vi "BNO055 Read AMG.vi"(8 "error in (no error)":errorcluster, 9 "BNO055 Config Options":T1={"I2C"={"Slave Address"=72, "Channel"=1}, "ADC"={"Channel"=4, "Expected Range (Programmable Gain Amplifier)"=0, "Sampling Mode"=1, "Sampling Rate"=4, "Comparator Mode"=1, "Comparator Polarity"=1, "Latching Comparator"=1, "Comparator Queue & Disable"=3}} {"ADC"."Comparator Queue & Disable" items=["Assert after one conversion", "Assert after two conversions", "Assert after four conversions", "Comparator disabled"]; "ADC"."Latching Comparator" items=["Non-latching", "Latching"]; "ADC"."Comparator Polarity" items=["Active Low", "Active High"]; "ADC"."Comparator Mode" items=["Traditional Comparator w/ hysteresis", "Window Comparator"]; "ADC"."Sampling Rate" items=["128SPS", "250SPS", "490SPS", "920SPS", "1600SPS", "2400SPS", "3300SPS"]; "ADC"."Sampling Mode" items=["Continuous Conversion", "Single-shot (Low Power)"]; "ADC"."Expected Range (Programmable Gain Amplifier)" items=["+/-6.144V", "+/-4.096V", "+/-2.048V", "+/-1.024V", "+/-0.512V", "+/-0.256V"]; "ADC"."Channel" items=["Differential: Ch 0&1", "Differential: Ch 0&3", "Differential: Ch 1&3", "Differential: Ch 2&3", "Single Ended: Ch 0", "Single Ended: Ch 1", "Single Ended: Ch 2", "Single Ended: Ch 3"]; "I2C"."Slave Address" format="%.0x"}, 11 "LINX Resource in":T3) -> (0 "error out":errorcluster, 1 "BNO055 Config Options":T1={"I2C"={"Slave Address"=72, "Channel"=1}, "ADC"={"Channel"=4, "Expected Range (Programmable Gain Amplifier)"=0, "Sampling Mode"=1, "Sampling Rate"=4, "Comparator Mode"=1, "Comparator Polarity"=1, "Latching Comparator"=1, "Comparator Queue & Disable"=3}} {"ADC"."Comparator Queue & Disable" items=["Assert after one conversion", "Assert after two conversions", "Assert after four conversions", "Comparator disabled"]; "ADC"."Latching Comparator" items=["Non-latching", "Latching"]; "ADC"."Comparator Polarity" items=["Active Low", "Active High"]; "ADC"."Comparator Mode" items=["Traditional Comparator w/ hysteresis", "Window Comparator"]; "ADC"."Sampling Rate" items=["128SPS", "250SPS", "490SPS", "920SPS", "1600SPS", "2400SPS", "3300SPS"]; "ADC"."Sampling Mode" items=["Continuous Conversion", "Single-shot (Low Power)"]; "ADC"."Expected Range (Programmable Gain Amplifier)" items=["+/-6.144V", "+/-4.096V", "+/-2.048V", "+/-1.024V", "+/-0.512V", "+/-0.256V"]; "ADC"."Channel" items=["Differential: Ch 0&1", "Differential: Ch 0&3", "Differential: Ch 1&3", "Differential: Ch 2&3", "Single Ended: Ch 0", "Single Ended: Ch 1", "Single Ended: Ch 2", "Single Ended: Ch 3"]; "I2C"."Slave Address" format="%.0x"}, 2 "IMU":T2 {"Gyroscope"."Z" scale=-45.0..45.0; "Gyroscope"."Y" scale=-45.0..45.0; "Gyroscope"."X" scale=-45.0..45.0; "Magnetometer"."Z" scale=-2500.0..2500.0; "Magnetometer"."Y" scale=-2500.0..2500.0; "Magnetometer"."X" scale=-2500.0..2500.0; "Accelerometer"."Z" scale=-5.0..5.0; "Accelerometer"."Y" scale=-5.0..5.0; "Accelerometer"."X" scale=-5.0..5.0}, 3 "LINX Resource":T3)   [LabVIEW 2014]
uses:
  <vilib>/MakerHub/LINX/Private/Type Defs/LINX Ref.ctl
  <vilib>/MakerHub/LINX/Private/Type Defs/Platform.ctl
  <vilib>/MakerHub/LINX/Private/Type Defs/Interface.ctl
  <vilib>/MakerHub/LINX/Private/Device/Type Defs/LINX Device Config.ctl
  <vilib>/MakerHub/LINX/Private/Device/Type Defs/TCP Config.ctl
  <vilib>/MakerHub/LINX/Private/Device/Type Defs/Channels.ctl
  BNO055 Config Options.ctl
  IMU Control.ctl
  <vilib>/MakerHub/LINX/LMH-LINX.lvlib
  <vilib>/MakerHub/LINX/Private/Device/Device.lvlib
panel:
  out "Array":u32[](array[numeric])
  out "Data out":u8[](array[numeric])
  out "Data":u8[](array[numeric])
  # "NOT DONE\nYET!"
  # "NOT DONE\nYET!"
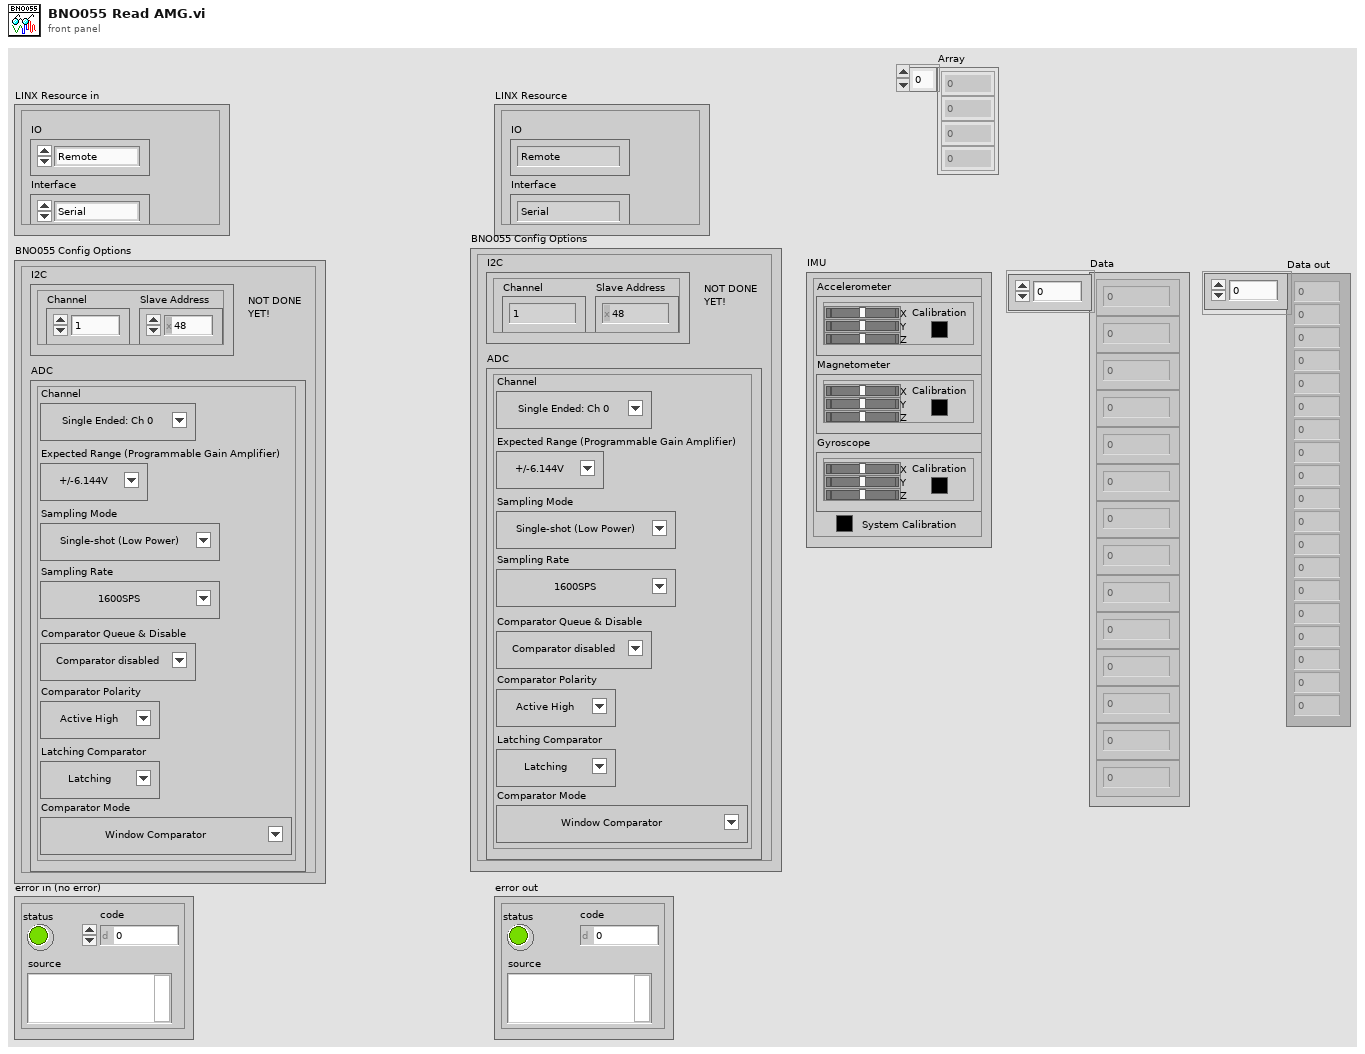
[diagram p1: front panel]
types:
  T1 = typedef "BNO055 Config Options.ctl" = cluster{"I2C":cluster{"Slave Address":u8, "Channel":u8}, "ADC":cluster{"Channel":u8, "Expected Range (Programmable Gain Amplifier)":u8, "Sampling Mode":u8, "Sampling Rate":u8, "Comparator Mode":u8, "Comparator Polarity":u8, "Latching Comparator":u8, "Comparator Queue & Disable":u8}}
  T2 = typedef "IMU Control.ctl" = cluster{"Accelerometer":cluster{"X":dbl, "Y":dbl, "Z":dbl, "Calibration":u32}, "Magnetometer":cluster{"X":dbl, "Y":dbl, "Z":dbl, "Calibration":u32}, "Gyroscope":cluster{"X":dbl, "Y":dbl, "Z":dbl, "Calibration":u32}, "System Calibration":u32}
  T3 = typedef "LMH-LINX.lvlib/LINX Ref.ctl" = cluster{"IO":T4, "Interface":T5, "LINX Device Config":T6}
  T4 = typedef "LMH-LINX.lvlib/Platform.ctl" = enum16{"Remote", "Local"}
  T5 = typedef "LMH-LINX.lvlib/Interface.ctl" = enum16{"Serial", "TCP"}
  T6 = typedef "LMH-LINX.lvlib/Device.lvlib/LINX Device Config.ctl" = cluster{"Interface":T5, "COM Port":refnum<visa-resource-name>, "TCP Configuration":T7, "Device Family":u8, "Device ID":u8, "Device Name":string, "TCP Ref":refnum<k5>, "Channels":T8}
  T7 = typedef "LMH-LINX.lvlib/Device.lvlib/TCP Config.ctl" = cluster{"IP Address":string, "Port":u16}
  T8 = typedef "LMH-LINX.lvlib/Channels.ctl" = cluster{"DI":u8[], "DO":u8[], "AI":u8[], "AO":u8[], "PWM":u8[], "QE":u8[], "UART":u8[], "I2C 2":u8[], "SPI":u8[], "CAN":u8[], "Servo":u8[], "AI Ref (V)":dbl, "AI Resolution (Bits)":u8, "AO Ref (V)":dbl, "AO Resolution (Bits)":u8}
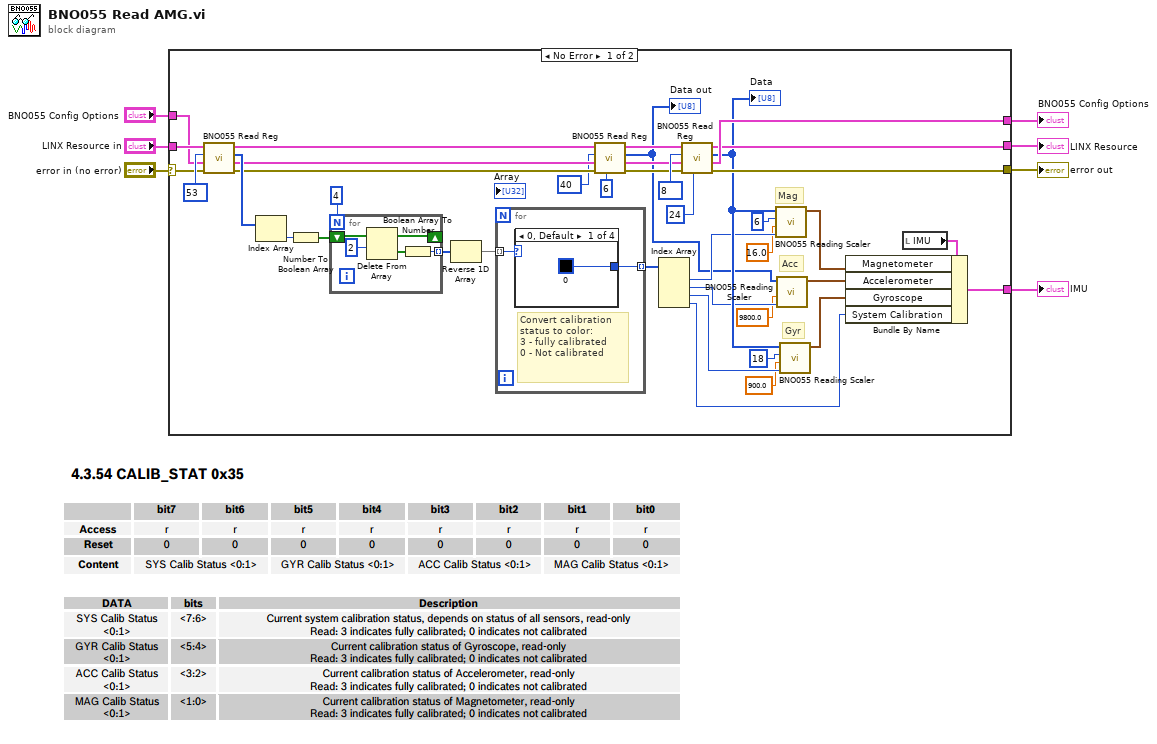
[diagram p0: block diagram]
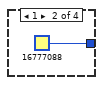
[diagram p2: hidden frame]
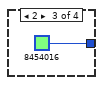
[diagram p3: hidden frame]
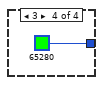
[diagram p4: hidden frame]
diagram:
  n1 = case shown="No Error" "error in (no error)" {
    selector: "error in (no error)" -> [w37 w60]
    tunnel: "LINX Resource in" -> [w38 w61]
    tunnel: "BNO055 Config Options" -> [w36 w59]
    tunnel: [w33 w61] -> w4
    tunnel: [w32 w60] -> w3
    tunnel: [w45 _] -> w1
    tunnel: [w47 w59] -> w2
    frame No Error {
      # "Gyr"
      # "Acc"
      # "Mag"
      n2 = call "BNO055 Read Reg.vi"("error in (no error)"=w37, "BNO055 Config Options"=w36, "Register"=u8 53 ("I2C Slave Address 2"), "LINX Resource in"=w38) -> ("error out"=w17:errorcluster, "BNO055 Config Options"=w16:T1, "Data out"=w39:u8[], "LINX Resource"=w15:T3)  [unwired: 4 in]
      n3 = Index Array(array=w39) -> (element=w44:u8)  [unwired: 1 in]
      n4 = Number To Boolean Array(number=w44) -> (Boolean array=w43:bool[])
      n5 = for {
        N: 4 -> [_]
        shift-right: [w50] -> _
        shift-left: w43 -> [w52]
        tunnel: [w48] -> w42 mode=indexing
        n6 = Delete From Array(array=w52, length=2) -> (deleted portion=w49:bool[], array with subset deleted=w50:bool[])  [unwired: 1 in]
        n7 = Boolean Array To Number(Boolean array=w49) -> (number=w48:u32)
      }
      n8 = Reverse 1D Array(array=w42) -> (reversed array=w8:u32[])
      n9 = for {
        tunnel: [w54] -> w46 mode=indexing
        tunnel: w8 -> [w53] mode=indexing
        # "Convert calibration status to color: \n3 - fully calibrated\n0 - Not calibrated"
        n10 = case shown="0, Default" w53 {
          tunnel: [u32 0 u32 16777088 u32 8454016 u32 65280] -> w54
          frame 0, Default {
          }
          frame 1 {
          }
          frame 2 {
          }
          frame 3 {
          }
        }
      }
      n11 = call "BNO055 Read Reg.vi"("Bytes To Read (1)"=u8 6 ("Bytes To Read"), "error in (no error)"=w17, "BNO055 Config Options"=w16, "Register"=u8 40 ("I2C Slave Address 2"), "LINX Resource in"=w15) -> ("error out"=w14:errorcluster, "BNO055 Config Options"=w13:T1, "Data out"=w9:u8[], "LINX Resource"=w12:T3)  [unwired: 3 in]
      "Data out" <- w9
      n12 = Index Array(array=w46) -> (element #1=w29:u32, element #2=w28:u32, element #3=w27:u32, element #4=w20:u32)  [unwired: 4 in]
      n13 = call "BNO055 Read Reg.vi"("Bytes To Read (1)"=u8 24 ("Bytes To Read"), "error in (no error)"=w14, "BNO055 Config Options"=w13, "Register"=u8 8 ("I2C Slave Address 2"), "LINX Resource in"=w12) -> ("error out"=w32:errorcluster, "BNO055 Config Options"=w47:T1, "Data out"=w30:u8[], "LINX Resource"=w33:T3)  [unwired: 3 in]
      "Data" <- w30
      n14 = call "BNO055 Reading Scaler.vi"("Calibration"=w29, "LSB Divider"=16.0, "index"=6, "AMG Reading"=w30) -> ("Sensor Cluster"=w26:cluster{"X":dbl, "Y":dbl, "Z":dbl, "Cal":u32})  [unwired: 7 in]
      n15 = call "BNO055 Reading Scaler.vi"("Calibration"=w28, "LSB Divider"=9800.0, "AMG Reading"=w9) -> ("Sensor Cluster"=w25:cluster{"X":dbl, "Y":dbl, "Z":dbl, "Cal":u32})  [unwired: 8 in]
      n16 = call "BNO055 Reading Scaler.vi"("Calibration"=w27, "LSB Divider"=900.0, "index"=18, "AMG Reading"=w30) -> ("Sensor Cluster"=w24:cluster{"X":dbl, "Y":dbl, "Z":dbl, "Cal":u32})  [unwired: 7 in]
      n17 = local read "IMU"() -> (w31:T2)
      n18 = Bundle By Name(cluster=w31, "Magnetometer"=w26, "Accelerometer"=w25, "Gyroscope"=w24, "System Calibration"=w20) -> (w45:T2)
    }
    frame Error {
    }
  }
  "error out" <- w3
  "LINX Resource" <- w4
  "IMU" <- w1
  "BNO055 Config Options" <- w2
